vi "test Buffer Offset.vi"(8 "error in (no error)":errorcluster, 11 "TestCase in":refnum<class "Configuration Tests.lvclass">) -> (0 "error out":errorcluster, 3 "TestCase out":refnum<class "Configuration Tests.lvclass">)   [LabVIEW 2017, in "Configuration Tests.lvclass"]
uses:
  Configuration Tests.lvclass
  Engine/Classes/Transfer/Transfer.lvclass
  <vilib>/NI/Memory Manager/Classes/Pointer/Pointer.lvclass/Pointer.ctl
  Engine/Classes/Transfer/Transfer.lvclass/Transfer.ctl
  <vilib>/NI/Memory Manager/Classes/Pointer/Public/New/New (8B).vi
  <vilib>/NI/Memory Manager/Classes/Pointer/Private/Allocate.vi
  <vilib>/NI/Memory Manager/Classes/Pointer/API/Accessors/Set Address.vi
  <vilib>/NI/Memory Manager/Classes/Pointer/API/Accessors/Set Size.vi
  <vilib>/NI/Memory Manager/Classes/Pointer/Private/Set Internal.vi
  Engine/Classes/Pointer/DBL Pointer.lvclass
  C:/Program Files (x86)/National Instruments/LabVIEW 2017/vi.lib/NI/Memory Manager/Classes/Pointer/Pointer.lvclass
  <vilib>/NI/Memory Manager/Classes/Pointer/Pointer.lvclass
  <vilib>/addons/_JKI Toolkits/VI Tester/TestCase.llb/TestCase.lvclass
  C:/Program Files (x86)/National Instruments/LabVIEW 2017/vi.lib/addons/_JKI Toolkits/VI Tester/TestCase.llb/TestCase.lvclass
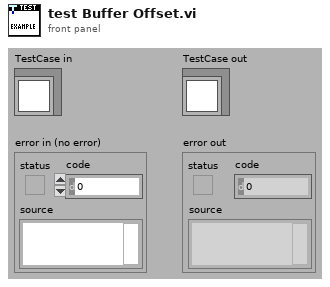
[diagram p1: front panel]
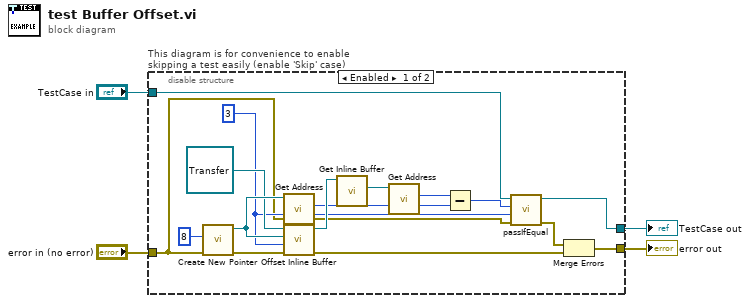
[diagram p0: block diagram]
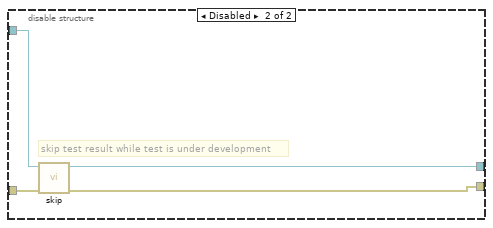
[diagram p2: hidden frame]
diagram:
  n1 = disable-structure "This diagram is for convenience to enable skipping a test easily (enable 'Skip' case)" shown="Enabled" {
    disable-tunnel: "TestCase in" -> [w14 w24]
    disable-tunnel: [w13 w22] -> w1
    disable-tunnel: [w8 w23] -> w3
    disable-tunnel: "error in (no error)" -> [w5 w21]
    frame Enabled {
      w9 = u64 3 ("group engine offset")
      n2 = call-poly <vilib>:"Create New Pointer.vi"("error in (no error)"=w5, "count (1)"=u64 8) -> ("error out"=w6:errorcluster, "Pointer"=w19:refnum<class "Pointer.lvclass">)  [unwired: 8 in]
      n3 = call <vilib>:"Get Address.vi"("Pointer in"=w19) -> ("address"=w11:u64)  [unwired: 9 in, 1 out]
      n4 = call "Offset Inline Buffer.vi"("error in (no error)"=w6, "group engine offset"=w9, "Engine Pointer"=w19, "Transfer in"=refnum<class "Transfer.lvclass"> refnum) -> ("error out"=w7:errorcluster, "Transfer out"=w17:refnum<class "Transfer.lvclass">)  [unwired: 6 in]
      n5 = call "Get Inline Buffer.vi"("Transfer in"=w17) -> ("Inline Buffer"=w16:refnum<class "DBL Pointer.lvclass">)  [unwired: 9 in, 1 out]
      n6 = call <vilib>:"Get Address.vi"("Pointer in"=w16) -> ("address"=w12:u64)  [unwired: 9 in, 1 out]
      n7 = Subtract(x=w12, y=w11) -> (x-y=w10:u64)
      n8 = call-dynamic "passIfEqual.vi"("error in (no error)"=w5, "y"=w9, "x"=w10, "TestCase in"=w14) -> ("error out"=w15:errorcluster, "TestCase out"=w13:refnum<class "Configuration Tests.lvclass">)  [unwired: 6 in]
      n9 = Merge Errors(w15, w7) -> (w8:errorcluster)
    }
    frame Disabled {
      # "skip test result while test is under development"
      n10 = call <vilib>:"skip.vi"("error in (no error)"=w21, "TestCase in"=w24) -> ("error out"=w23:errorcluster, "TestCase out"=w22:refnum<class "Configuration Tests.lvclass">)  [unwired: 8 in]
    }
  }
  "error out" <- w3
  "TestCase out" <- w1
